vi "LockControl.vi"   [LabVIEW 2018]
uses:
  ClimbLockEnum.ctl
  <vilib>/Rock Robotics/WPI/Utilities/WPI_GetSetVariantRefNum.vi
types:
  T1 = typedef "WPI_JoystickDevRef.ctl" = cluster{"Device":T2}
  T2 = typedef "WPI_JoystickDeviceEnum.ctl" = enum16{"USB 0", "USB 1", "USB 2", "USB 3", "USB 4", "USB 5"}
  T3 = typedef "ClimbLockEnum.ctl" = enum16{"Both Locked", "Both Unlocked"}
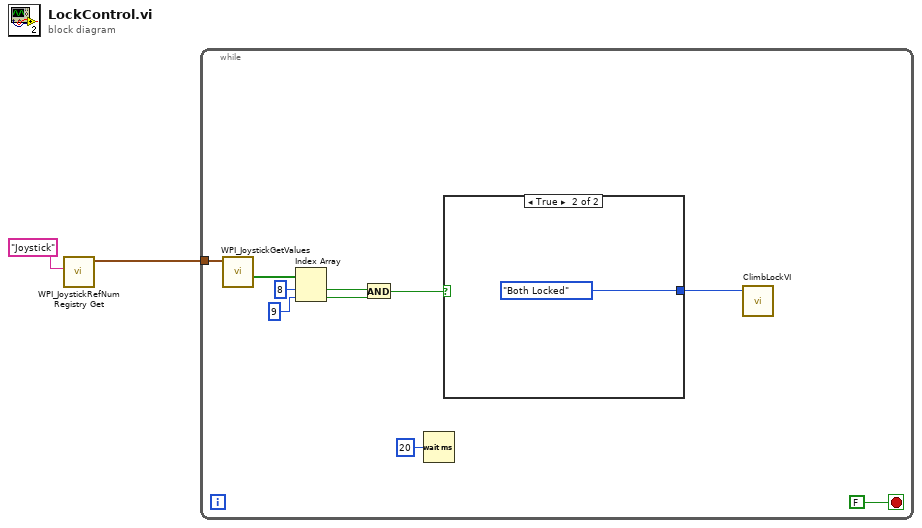
[diagram p0: block diagram]
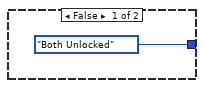
[diagram p2: hidden frame]
diagram:
  n1 = call <vilib>:"WPI_JoystickRefNum Registry Get.vi"("refnum name"="Joystick") -> ("JoystickDevRef"=w2:T1)  [unwired: 9 in, 1 out]
  n2 = while {
    tunnel: w2 -> [w12]
    stop <- FALSE stop-if-true
    n3 = call <vilib>:"WPI_JoystickGetValues.vi"("JoystickDevRef"=w12) -> ("Buttons"=w11:bool[])  [unwired: 6 in, 4 out]
    n4 = Index Array(array=w11, index #1=8 ("index"), index #2=9 ("index")) -> (element #1=w8:bool, element #2=w7:bool)
    n5 = And(x=w8, y=w7) -> (x .and. y?=w6:bool)
    n6 = Wait (ms)(milliseconds to wait=u32 20) -> ()  [unwired: 1 out]
    n7 = case shown="True" w6 {
      tunnel: [ClimbLockEnum."Both Unlocked" ("LockStates") ClimbLockEnum."Both Locked" ("LockStates")] -> w5
      frame False {
      }
      frame True {
      }
    }
    n8 = call "ClimbLockVI.vi"("LockStates"=w5) -> ()  [unwired: 11 in]
  }
